vi "Aggiungi acquisizione.vi"(10 "Nuova riga":string[](array[string]), 11 "Dati in":string[][](array[string])) -> (2 "riga":string[](array[string]), 3 "Dati out":string[][](array[string]))   [LabVIEW 2019]
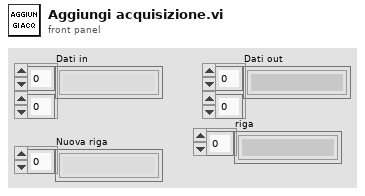
[diagram p1: front panel]
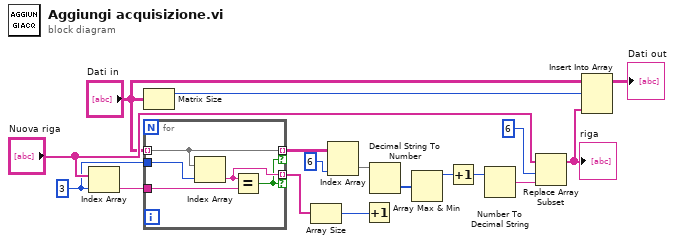
[diagram p0: block diagram]
diagram:
  w11 = 3 ("index")
  n1 = Index Array(array="Nuova riga", index=w11) -> (element=w12:string)
  n2 = Matrix Size(0:"Dati in") -> (1:w8:i32)  [unwired: 1 out]
  n3 = for {
    tunnel: "Dati in" -> [w19] mode=indexing
    tunnel: w11 -> [w22]
    tunnel: w12 -> [w20]
    tunnel: [w21] -> w7 mode=indexing if=w18
    tunnel: [w19] -> w5 mode=indexing if=w18
    n4 = Index Array(array=w19, index=w22) -> (element=w21:string)
    n5 = Equal?(x=w21, y=w20) -> (x = y?=w18:bool)
  }
  n6 = Array Size(array=w7) -> (size(s)=w13:i32)
  n7 = Index Array(array=w5, index (col)=6 ("index")) -> (element=w6:string[])  [unwired: 1 in]
  n8 = Increment(x=w13) -> ()  [unwired: 1 out]
  n9 = Decimal String To Number(string=w6) -> (number=w3:i32[])  [unwired: 2 in, 1 out]
  n10 = Array Max & Min(array=w3) -> (max value=w2:i32)  [unwired: 3 out]
  n11 = Increment(x=w2) -> (x+1=w1:i32)
  n12 = Number To Decimal String(number=w1) -> (decimal integer string=w16:string)  [unwired: 1 in]
  n13 = Replace Array Subset(array="Nuova riga", new element=w16, index=6) -> (w17:string[])
  "riga" <- w17
  n14 = Insert Into Array(array="Dati in", index (row)=w8, new element=w17) -> (→"Dati out":string[][])  [unwired: 1 in]
